vi "Truncate Idle Time.vi"(8 "error in (no error)":errorcluster, 10 "Digital Waveform":digitalwaveform(waveform)={"t0"=timestamp(0 s since 1904-01-01), "dt"=1.0, "Y"={"transitions"=[], "data"=[]}}, 11 "Truncate Waveform Settings":T1) -> (0 "error out":errorcluster, 2 "Digital Waveform out":digitalwaveform(waveform)={"t0"=timestamp(0 s since 1904-01-01), "dt"=1.0, "Y"={"transitions"=[], "data"=[]}})   [LabVIEW 2016]
uses:
  Typedefs/Truncate Waveform Settings.ctl
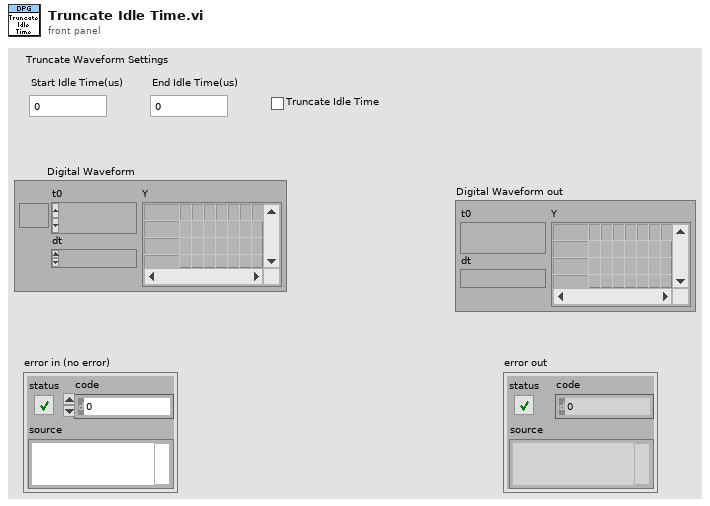
[diagram p1: front panel]
types:
  T1 = typedef "Truncate Waveform Settings.ctl" = cluster{"Truncate Idle Time":bool, "Start Idle Time(us)":dbl, "End Idle Time(us)":dbl}
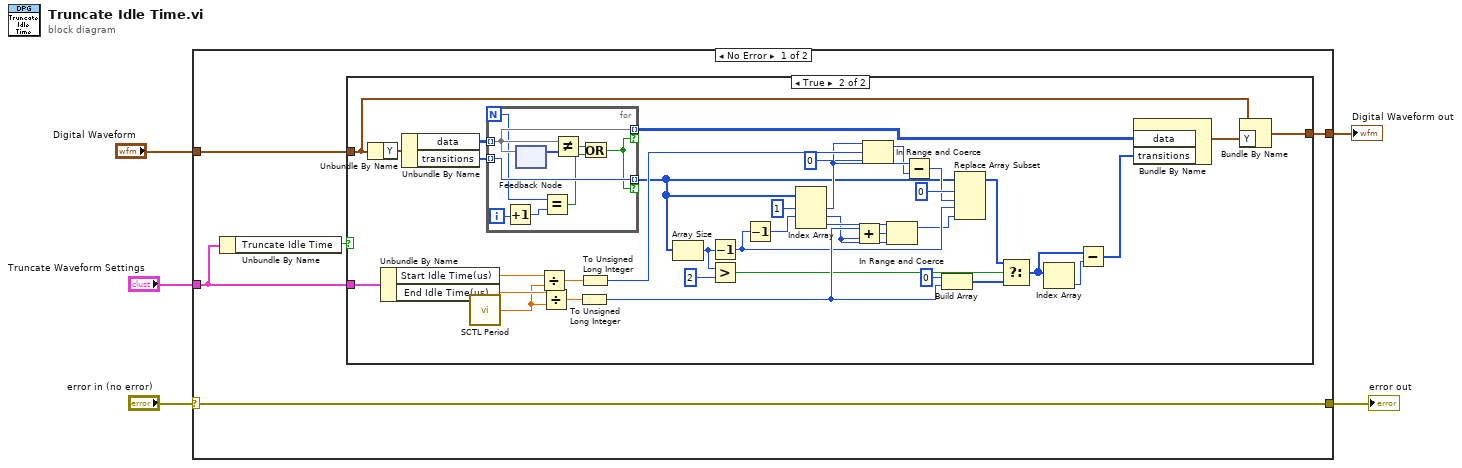
[diagram p0: block diagram]
diagram:
  n1 = case shown="No Error" "error in (no error)" {
    selector: "error in (no error)" -> [w10 w58]
    tunnel: [w10 w58] -> w4
    tunnel: "Digital Waveform" -> [w9 w59]
    tunnel: "Truncate Waveform Settings" -> [w8 _]
    tunnel: [w6 w59] -> w1
    frame No Error {
      n2 = Unbundle By Name(w8) -> ("Truncate Idle Time"=w7:bool)
      n3 = case shown="True" w7 {
        tunnel: w9 -> [w11 w13]
        tunnel: w8 -> [_ w45]
        tunnel: [w11 w12] -> w6
        frame False {
        }
        frame True {
          n4 = Unbundle By Name(w13) -> ("Y"=w48:digitaldata)
          n5 = Unbundle By Name(w45) -> ("Start Idle Time(us)"=w44:dbl, "End Idle Time(us)"=w43:dbl)
          n6 = Unbundle By Name(w48) -> ("data"=w47:u8[][], "transitions"=w46:u32[])
          n7 = call "SCTL Period.vi"() -> ("Clock Period(micro second)"=w42:dbl)  [unwired: 15 in]
          n8 = for {
            N -> [w51]
            tunnel: w47 -> [w56] mode=indexing
            tunnel: w46 -> [w55] mode=indexing
            tunnel: [w56] -> w16 mode=indexing if=w50
            tunnel: [w55] -> w19 mode=indexing if=w50
            i -> [w53]
            n9 = Increment(x=w53) -> (x+1=w52:i32)
            n10 = feedback-in #1(w56) -> ()
            n11 = feedback #1() -> (w57:u8[])  [unwired: 1 in]
            n12 = Equal?(x=w51, y=w52) -> (x = y?=w49:bool)
            n13 = Not Equal?(x=w56, y=w57) -> (x != y?=w54:bool)
            n14 = Or(x=w54, y=w49) -> (x .or. y?=w50:bool)
          }
          n15 = Divide(x=w44, y=w42) -> (x/y=w41:dbl)
          n16 = Divide(x=w43, y=w42) -> (x/y=w40:dbl)
          n17 = To Unsigned Long Integer(number=w40) -> (unsigned 32bit integer=w38:u32)
          n18 = To Unsigned Long Integer(number=w41) -> (unsigned 32bit integer=w39:u32)
          n19 = Array Size(array=w19) -> (size(s)=w33:i32)
          n20 = Decrement(x=w33) -> (x-1=w34:i32)
          n21 = Greater?(x=w33, y=2) -> (0:w31:bool)
          n22 = Decrement(x=w34) -> (x-1=w35:i32)
          n23 = Index Array(array=w19, index #1=1 ("index"), index #2=w35) -> (element #1=w29:u32, element #2=w22:u32, element #3=w25:u32)  [unwired: 1 in]
          n24 = Add(x=w38, y=w22) -> (x+y=w24:u32)
          n25 = In Range and Coerce(upper limit=w29, x=w39, lower limit=u32 0) -> (coerced(x)=w28:u32)  [unwired: 1 out]
          n26 = In Range and Coerce(upper limit=w25, x=w24, lower limit=w22) -> (coerced(x)=w23:u32)  [unwired: 1 out]
          n27 = Subtract(x=w29, y=w28) -> (x-y=w27:u32)
          n28 = Build Array(u32 0 ("element"), w38) -> (w20:u32[])
          n29 = Replace Array Subset(array=w19, new element #1=w27, index #1=0 ("index"), new element #2=w23, index #2=w34) -> (w30:u32[])
          n30 = Select(t=w30, s=w31, f=w20) -> (s? t:f=w17:u32[])
          n31 = Index Array(array=w17) -> (element=w18:u32)  [unwired: 1 in]
          n32 = Subtract(x=w17, y=w18) -> (x-y=w15:u32[])
          n33 = Bundle By Name("data"=w16, "transitions"=w15) -> (w14:digitaldata)  [unwired: 1 in]
          n34 = Bundle By Name(cluster=w13, "Y"=w14) -> (w12:digitalwaveform)
        }
      }
    }
    frame Error {
    }
  }
  "error out" <- w4
  "Digital Waveform out" <- w1
